vi "Generate_utils_script.vi"(8 "error in (no error)":errorcluster, 11 "Path":path) -> (0 "error out":errorcluster)   [LabVIEW 2018, in "Python.lvclass"]
uses:
  Python.lvclass
  <userlib>/_OpenG.lib/file/file.llb/File Exists - Scalar__ogtk.vi
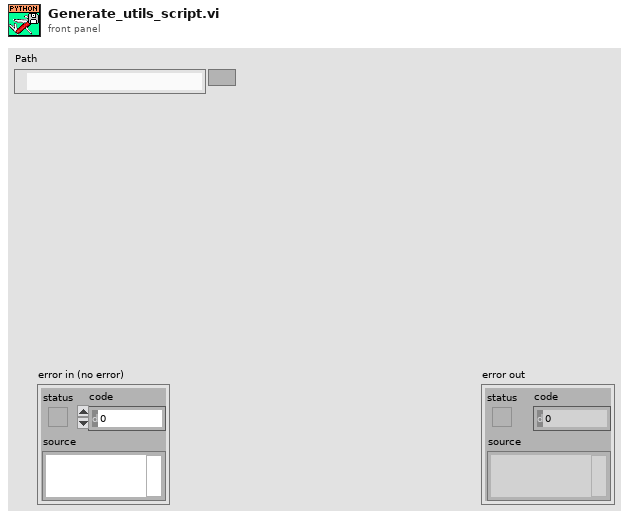
[diagram p1: front panel]
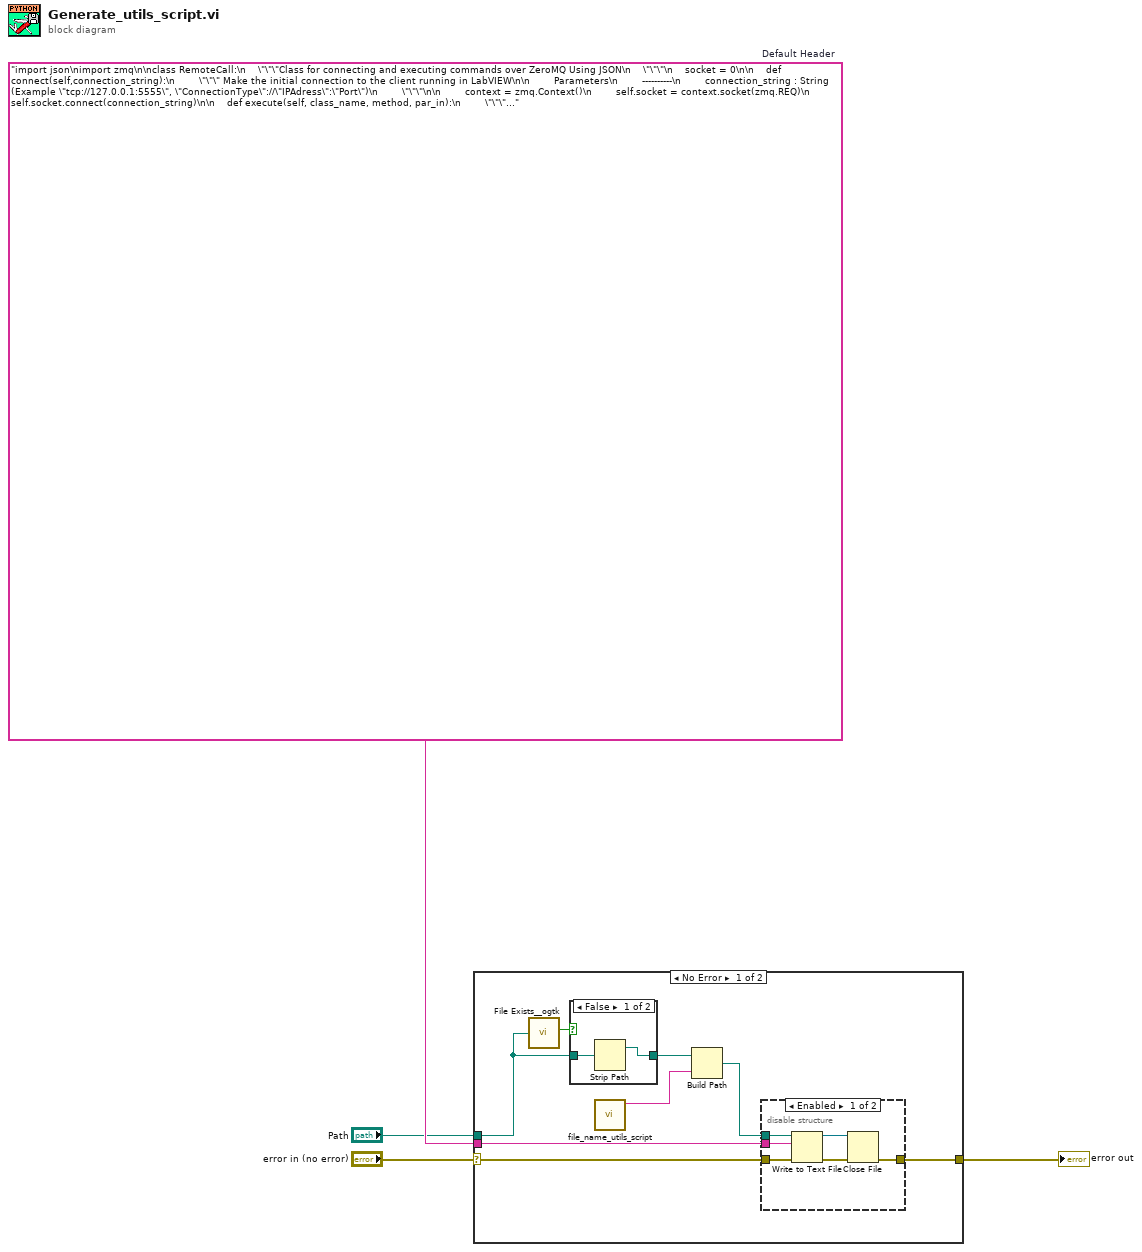
[diagram p0: block diagram]
diagram:
  w2 = "import json\nimport zmq\n\nclass RemoteCall:\n    \"\"\"Class for connecting and executing commands over ZeroMQ Using JSON\n    \"\"\"\n    socket = 0\n\n    def connect(self,connection_string):\n        \"\"\" Make the initial connection to the client running in LabVIEW\n\n        Parameters\n        ----------\n        connection_string : String (Example \"tcp://127.0.0.1:5555\", \"ConnectionType\"://\"IPAdress\":\"Port\")\n        \"\"\"\n\n        context = zmq.Context()\n        self.socket = context.socket(zmq.REQ)\n        self.socket.connect(connection_string)\n\n    def execute(self, class_name, method, par_in):\n        \"\"\" Execute the Method by serializing inputs sending it over, and deserializing the result\n        \"\"\"\n        data_2_send = \"{ \\\"Command\\\":\\\"Execute\\\" }\\x17{\\\"ClassLabel\\\":\\\"%s\\\",\\\"Method\\\":\\\"%s\\\"}\\x17%s\" % (class_name, method, json.dumps({\"In\": par_in}))\n        self.socket.send_string (data_2_send)\n        message = self.socket.recv()\n        parts = message.split(chr(0x17).encode())\n        return json.loads(parts[1]), json.loads(parts[0])\n\nclass LabVIEWerror(Exception):\n    \"\"\"Base class for all LabVIEW errors\n\n    Attributes\n    ----------\n    code: error code for testing which error happend\n    source: source of the error\n    \"\"\"\n    def __init__(self, *args: object) -> None:\n        self.code = self.args[0]\n        self.source = self.args[1]\n        super().__init__(*args)\n\n    def __str__(self) -> str:\n        return f\"LabVIEW Error with code: {self.code} source: {self.source}\"\n"  # Default Header
  n1 = case shown="No Error" "error in (no error)" {
    selector: "error in (no error)" -> [w12 w23]
    tunnel: [w11 w23] -> w3
    tunnel: w2 -> [w10 _]
    tunnel: "Path" -> [w8 _]
    frame No Error {
      n2 = call-poly <userlib>:"File Exists__ogtk.vi"("file path"=w8) -> ("is directory"=w9:bool)  [unwired: 6 in, 1 out]
      n3 = case shown="False" w9 {
        tunnel: w8 -> [w21 w22]
        tunnel: [w20 w22] -> w7
        frame False {
          n4 = Strip Path(path=w21) -> (stripped path=w20:path)  [unwired: 1 out]
        }
        frame True {
        }
      }
      n5 = call "file_name_utils_script.vi"() -> ("file_name_utilities_script"=w5:string)  [unwired: 10 in, 1 out]
      n6 = Build Path(base path=w7, name or relative path=w5) -> (appended path=w6:path)
      n7 = disable-structure shown="Enabled" {
        disable-tunnel: w12 -> [w17 w19]
        disable-tunnel: [w16 w19] -> w11
        disable-tunnel: w10 -> [w14 _]
        disable-tunnel: w6 -> [w13 _]
        frame Enabled {
          n8 = Write to Text File(file (use dialog)=w13, text=w14, error in=w17) -> (refnum out=w15:refnum<file>, error out=w18:errorcluster)  [unwired: 1 in, 1 out]
          n9 = Close File(refnum=w15, error in=w18) -> (error out=w16:errorcluster)  [unwired: 1 out]
        }
        frame Disabled {
        }
      }
    }
    frame Error {
    }
  }
  "error out" <- w3
